vi "PublishInitPos.vi"(4 "AxisNumber":u8, 6 "ActPos":dbl, 8 "error in (no error)":errorcluster, 11 "CS++Motor in":refnum<class "CS++Motor.lvclass">) -> (0 "error out":errorcluster, 3 "CS++Motor out":refnum<class "CS++Motor.lvclass">)   [LabVIEW 2016, in "CS++Motor.lvlib" / "CS++Motor.lvclass"]
doc: "This VI publishes the Act and Set Positions during a reset cmd."
uses:
  CS++Motor.lvclass
  PV-Enum-n.ctl
  CSPP_Core/Classes/CS++ProcessVariables/ProcessVariable/PV.lvclass
  CS++Motor.lvclass/CS++Motor.ctl
  CSPP_Core/Classes/CS++ProcessVariables/ProcessVariable/PV.lvclass/PV.ctl
  CSPP_Core/Classes/CS++ProcessVariables/ProcessVariable/Write Data.vi
  CSPP_Core/Classes/CS++ProcessVariables/ProcessVariable/Write Timestamp.vi
  CSPP_Core/Classes/CS++ProcessVariables/ProcessVariable/Write Quality.vi
  CSPP_Core/Classes/CS++ProcessVariables/ProcessVariable/Write status.vi
  CSPP_Core/Classes/CS++ProcessVariables/PVConnection/PVConnection.lvclass
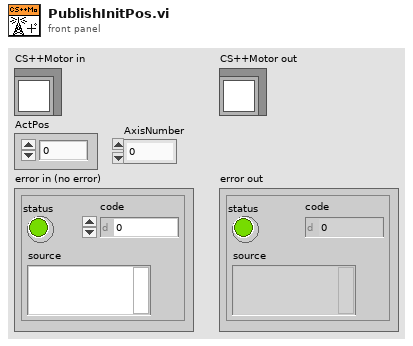
[diagram p1: front panel]
types:
  T1 = typedef "CS++Motor.lvlib/CS++Motor.lvclass/PV-Enum-n.ctl" = enum16{"PhysicalName", "unit", "ActPosition", "SetPosition", "RawSetPosition", "StartVelocity", "StopVelocity", "Acceleration", "RangeMin", "RangeMax", "Scaling", "ScalingOffset", "RangeRefError", "LogicalPositionArray", "NoOfCommands"}
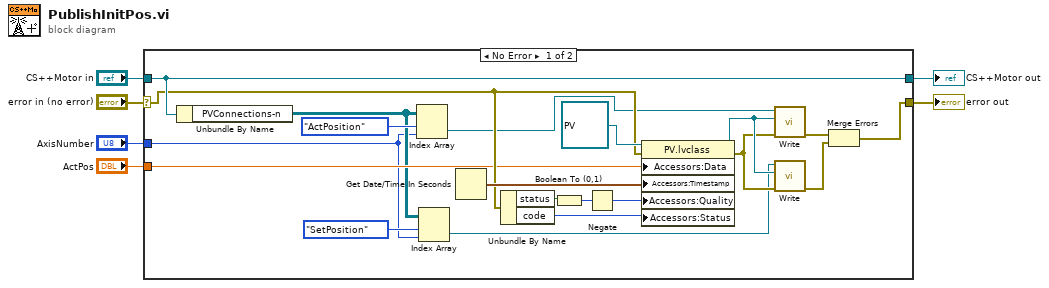
[diagram p0: block diagram]
diagram:
  n1 = case shown="No Error" "error in (no error)" {
    selector: "error in (no error)" -> [w18 w28]
    tunnel: [w7 w28] -> w5
    tunnel: [w26 w27] -> w2
    tunnel: "CS++Motor in" -> [w26 w27]
    tunnel: "ActPos" -> [w17 _]
    tunnel: "AxisNumber" -> [w14 _]
    frame No Error {
      n2 = Unbundle By Name(w26) -> ("PVConnections-n"=w15:refnum<class "PVConnection.lvclass">[][])
      n3 = Index Array(array=w15, index (row)=PV-Enum-n."ActPosition" ("PV-Enum-n"), index (col)=w14) -> (element=w13:refnum<class "PVConnection.lvclass">)
      n4 = Index Array(array=w15, index (row)=PV-Enum-n."SetPosition" ("PV-Enum-n"), index (col)=w14) -> (element=w10:refnum<class "PVConnection.lvclass">)
      n5 = Get Date/Time In Seconds() -> (seconds since 1Jan1904=w19:timestamp)
      n6 = Unbundle By Name(w18) -> ("status"=w23:bool, "code"=w22:i32)
      n7 = Boolean To (0,1)(Boolean=w23) -> (0, 1=w21:i16)
      n8 = Negate(x=w21) -> (-x=w24:i16)
      n9 = property class="PV.lvclass"(reference=refnum<class "PV.lvclass"> refnum ("PV"), error in=w18, "Accessors:Data"=w17, "Accessors:Timestamp"=w19, "Accessors:Quality"=w24, "Accessors:Status"=w22) -> (reference out=w12:refnum<class "PV.lvclass">, error out=w11:errorcluster)
      n10 = call "Write.vi"("error in (no error)"=w11, "PV"=w12, "PVConnection in"=w13) -> ("error out"=w9:errorcluster)  [unwired: 7 in, 1 out]
      n11 = call "Write.vi"("error in (no error)"=w11, "PV"=w12, "PVConnection in"=w10) -> ("error out"=w8:errorcluster)  [unwired: 7 in, 1 out]
      n12 = Merge Errors(w9, w8) -> (w7:errorcluster)
    }
    frame Error {
    }
  }
  "error out" <- w5
  "CS++Motor out" <- w2
